vi "writeBoolean.vi"(8 "error in (no error)":errorcluster, 10 "Data":bool, 11 "IBooleanControl in":refnum<class "IBooleanControl.lvclass">) -> (0 "error out":errorcluster, 3 "IBooleanControl out":refnum<class "IBooleanControl.lvclass">)   [LabVIEW 2015, in "RTFPGA.lvlib" / "IBooleanControl.lvclass"]
uses:
  IBooleanControl.lvclass
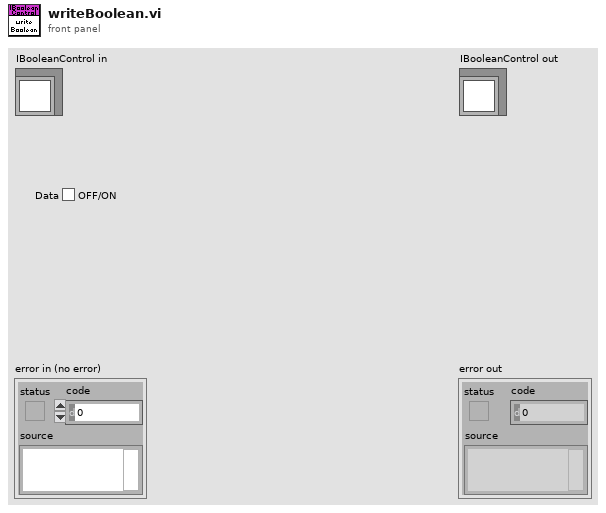
[diagram p1: front panel]
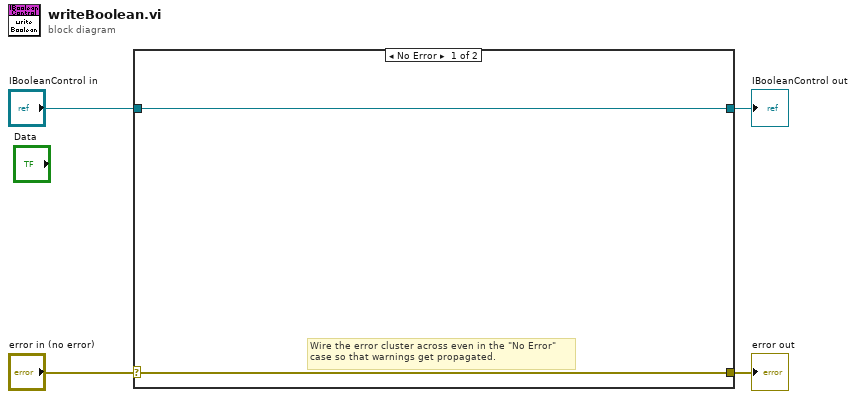
[diagram p0: block diagram]
diagram:
  n1 = case shown="No Error" "error in (no error)" {
    selector: "error in (no error)" -> [w5 w8]
    tunnel: [w5 w8] -> w3
    tunnel: [w6 w7] -> w1
    tunnel: "IBooleanControl in" -> [w6 w7]
    frame No Error {
      # "Wire the error cluster across even in the \"No Error\"\ncase so that warnings get propagated."
    }
    frame Error {
    }
  }
  "error out" <- w3
  "IBooleanControl out" <- w1
